vi "Groups for Channels.vi"(8 "error in (no error)":errorcluster, 10 "Channels":string[](array[string]), 11 "VolatusAPI in":refnum<class "VolatusAPI.lvclass">) -> (0 "error out":errorcluster, 1 "Channels per Group":cluster{"Channels":string[]}[](array[cluster]), 2 "Groups":string[](array[string]), 3 "VolatusAPI out":refnum<class "VolatusAPI.lvclass">)   [LabVIEW 2020, in "Volatus.lvlib" / "VolatusAPI.lvclass"]
uses:
  VolatusAPI.lvclass
  VolatusAPI.lvclass/VolatusAPI.ctl
  <vilib>/Utility/miscctls.llb/LVMapReplaceAction.ctl
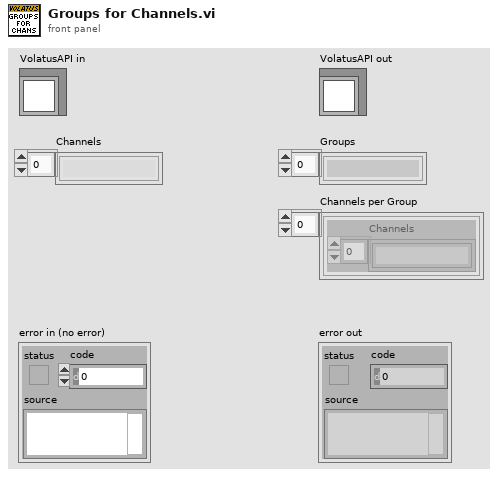
[diagram p1: front panel]
types:
  T1 = typedef "LVMapReplaceAction.ctl" = enum32{"Modify Entry only if found", "Add or Modify Entry", "Delete Entry"}
  T2 = typedef "VectoConfig.lvlib/Channel Info.ctl" = cluster{"Name":string, "Group":string, "Owning Node":string, "Owning Task":string, "Resource":string}
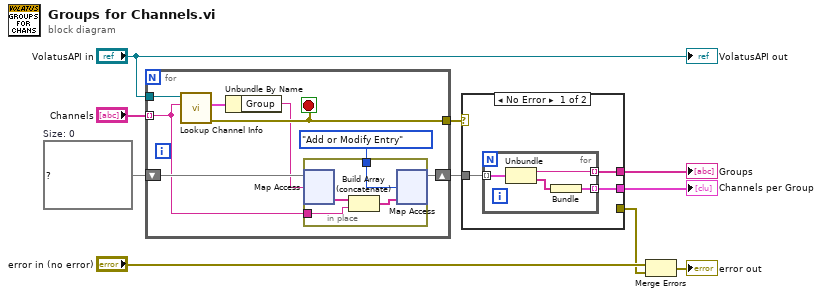
[diagram p0: block diagram]
diagram:
  w6 = map{string, string[]} {}  # Size: 0
  n1 = for {
    tunnel: "Channels" -> [w13] mode=indexing
    tunnel: "VolatusAPI in" -> [w18]
    shift-right: [w11] -> w5
    shift-left: w6 -> [w15]
    tunnel: [w16] -> w4
    stop <- w16 stop-if-true
    n2 = call "Lookup Channel Info.vi"("Channel Name"=w13, "VolatusAPI in"=w18) -> ("error out"=w16:errorcluster, "Channel Info"=w17:T2)  [unwired: 6 in, 2 out]
    n3 = Unbundle By Name(w17) -> ("Group"=w14:string)
    n4 = in-place {
      in-place-border: w13 -> [w21]
      in-place-border: LVMapReplaceAction."Add or Modify Entry" ("action") -> [w19]
      n5 = in-place-map #1(w15, w14) -> (w22:string[])  [unwired: 1 in, 1 out]
      n6 = Build Array (concatenate)(w22, w21) -> (w20:string[])
      n7 = in-place-map #1(w20, w19) -> (w11:map{string, string[]})  [unwired: 2 out]
    }
  }
  n8 = case shown="No Error" w4 {
    selector: w4 -> [_ w30]
    tunnel: w5 -> [w25 _]
    tunnel: [w24 _] -> w3
    tunnel: [w23 _] -> w2
    tunnel: [_ w30] -> w1
    frame No Error {
      n9 = for {
        tunnel: w25 -> [w29] mode=indexing
        tunnel: [w27] -> w24 mode=indexing
        tunnel: [w26] -> w23 mode=indexing
        n10 = Unbundle(w29) -> (w26:string, "Channels"=w28:string[])
        n11 = Bundle("Channels"=w28) -> (w27:cluster{"Channels":string[]})  [unwired: 1 in]
      }
    }
    frame Error {
    }
  }
  "Groups" <- w2
  "Channels per Group" <- w3
  n12 = Merge Errors("error in (no error)", w1) -> (→"error out":errorcluster)
  "VolatusAPI out" <- "VolatusAPI in"
